vi "Import Hardware Config.vi"(0 "Configuration file":path, 5 "Import Mode":u32(ring)=2097152 items=["merge"=0, "replace all"=1048576, "preserve existing"=2097152], 11 "error in (no error)":errorcluster) -> (15 "error out":errorcluster)   [LabVIEW 2021]
doc: "Imports the data from selected configuration file to NI-Max"
uses:
  <vilib>/nisyscfg/Close (System).vi
  <vilib>/nisyscfg/nisyscfg.lvlib
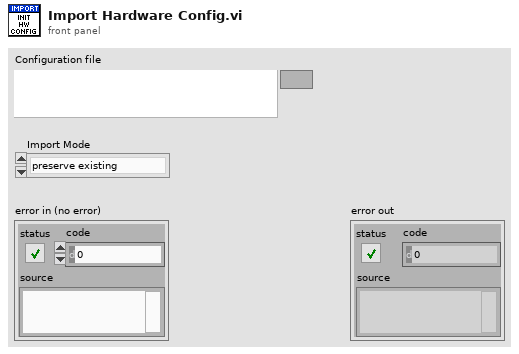
[diagram p1: front panel]
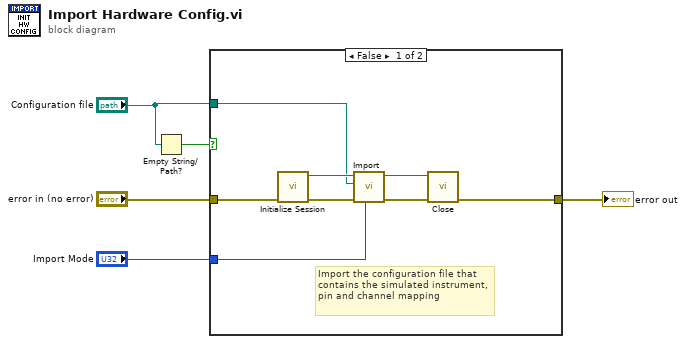
[diagram p0: block diagram]
diagram:
  n1 = Empty String/Path?(string/path="Configuration file") -> (empty?=w2:bool)
  n2 = case shown="False" w2 {
    tunnel: "error in (no error)" -> [w13 w14]
    tunnel: [w12 w14] -> w4
    tunnel: "Configuration file" -> [w7 _]
    tunnel: "Import Mode" -> [w6 _]
    frame False {
      # "Import the configuration file that contains the simulated instrument, pin and channel mapping"
      n3 = call <vilib>:"Initialize Session.vi"("error in (no error)"=w13) -> ("error out"=w11:errorcluster, "Session out"=w9:refnum<k21>)  [unwired: 9 in]
      n4 = call <vilib>:"Import.vi"("Import Mode"=w6, "error in (no error)"=w11, "Source File"=w7, "Session in"=w9) -> ("error out"=w10:errorcluster, "Session out"=w8:refnum<k21>)  [unwired: 5 in, 1 out]
      n5 = call-poly <vilib>:"Close.vi"("error in (no error)"=w10, "Session in"=w8) -> ("error out"=w12:errorcluster)  [unwired: 9 in]
    }
    frame True {
    }
  }
  "error out" <- w4
